vi "Example.vi"() -> ()   [LabVIEW 2018]
uses:
  Data Def/IT8800-Setting.ctl
panel:
  in  "Range Type":u16(ring) items=["Current", "Voltage", "Power", "Conductance"]
  out "Range":u16(ring)=2 items=["Low", "Medium", "High"]
  in  "Tracer":bool
  in  "Apply":bool
  in  "Value":dbl=5.0
  in  "Operation Mode":enum16{"CC", "CV", "CP"}(ring)
  out "Input?":bool
  in  "Stop Load":bool
  in  "Apply Load":bool
  out "Chart":T1(graph)={"Voltage (Volts)"=-1.0, "Power (Watts)"=-1.0, "Current (Amps)"=-1.0}
  out "Stop?":bool
  in  "IT8800 Setting In In":T2={"VISA Resource Name"="COM4", "Baud Rate"=9600, "Stop Bits"=10, "Wait For Read(ms)"=10} {"Stop Bits" items=["1.0"=10, "2.0"=20]; "Baud Rate" items=["2400"=2400, "4800"=4800, "9600"=9600, "19200"=19200]}
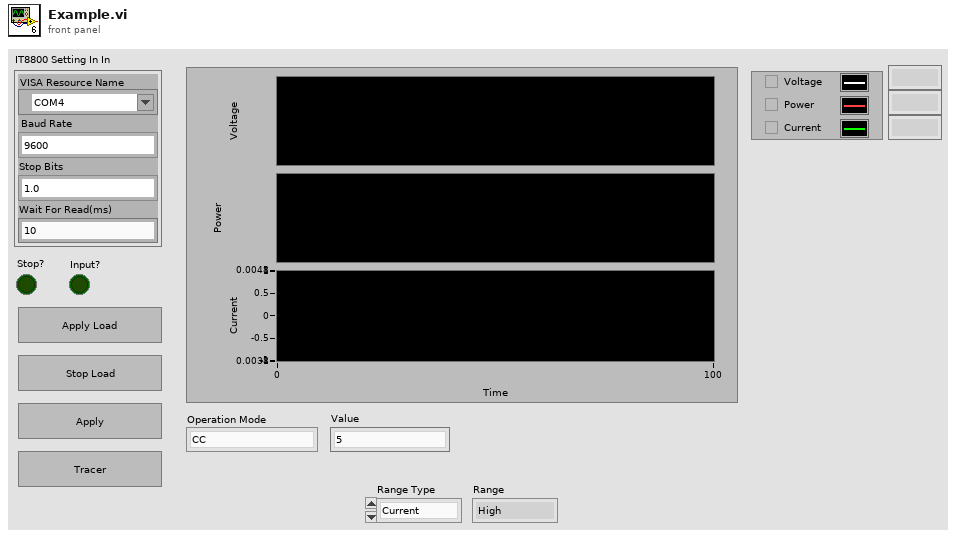
[diagram p1: front panel]
types:
  T1 = cluster{"Voltage (Volts)":dbl, "Power (Watts)":dbl, "Current (Amps)":dbl}
  T2 = typedef "IT8800-Setting.ctl" = cluster{"VISA Resource Name":refnum<visa-resource-name>, "Baud Rate":u32, "Stop Bits":u16, "Wait For Read(ms)":u32}
  T3 = typedef "IT8800-Measurement Data.ctl" = cluster{"Current (Amps)":dbl, "Power (Watts)":dbl, "Voltage (Volts)":dbl, "Elapsed Time (Sec) ":dbl}
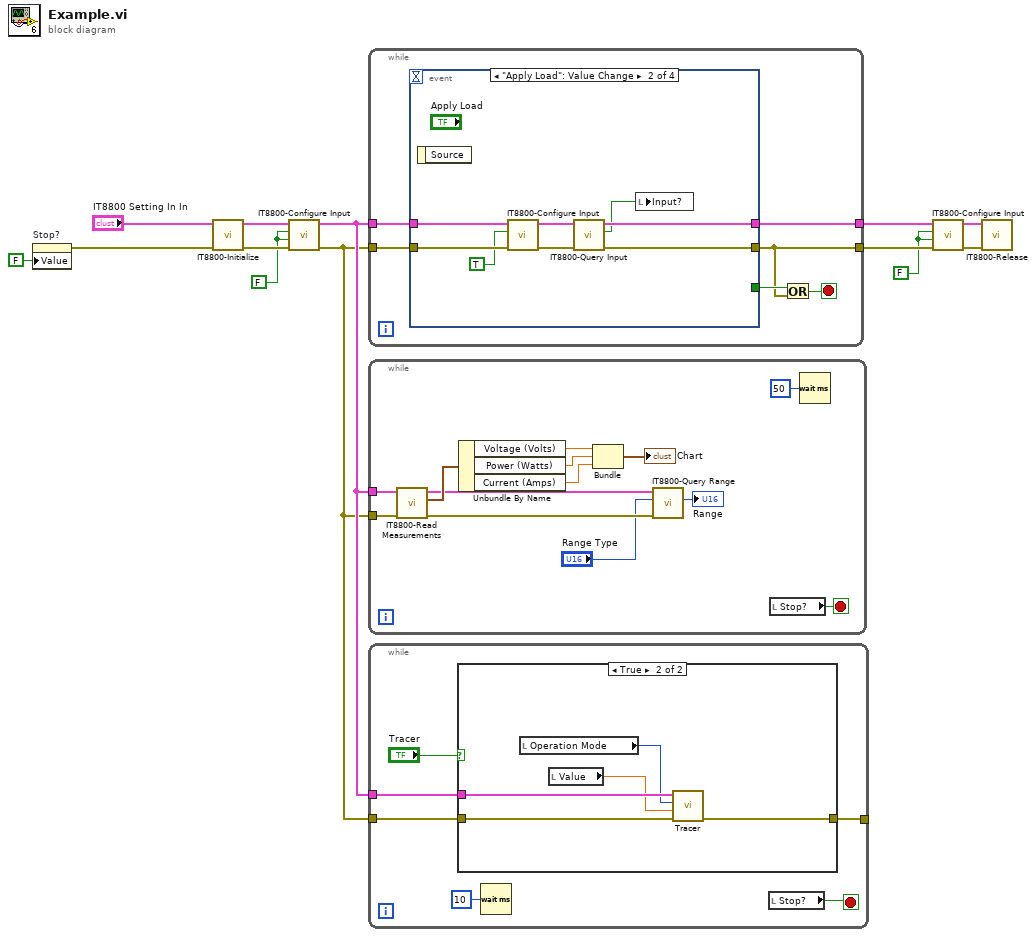
[diagram p0: block diagram]
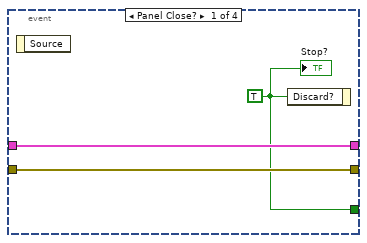
[diagram p3: hidden frame]
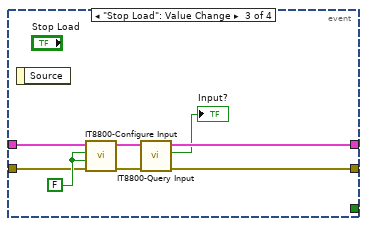
[diagram p4: hidden frame]
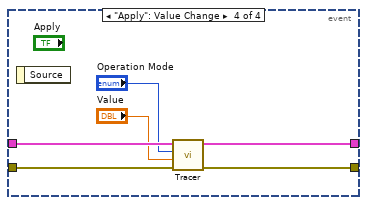
[diagram p5: hidden frame]
diagram:
  w5 = FALSE ("Enable Input")
  w10 = FALSE ("Enable Input")
  n1 = property on="Stop?" class="Bool (strict)"("Value"=FALSE ("Stop?")) -> (error out=w4:errorcluster)  [unwired: 2 in, 1 out]
  n2 = call "IT8800-Initialize.vi"("error in (no error)"=w4, "ITech Setting In"="IT8800 Setting In In") -> ("error out"=w11:errorcluster, "IT8800 Setting In Out"=w12:T2)  [unwired: 8 in]
  n3 = call "IT8800-Configure Input.vi"("error in"=w11, "Enable Input Short"=w10, "Enable Input"=w10, "IT8800 Setting In In"=w12) -> ("error out"=w1:errorcluster, "IT8800 Setting In Out"=w2:T2)  [unwired: 6 in]
  n4 = while {
    tunnel: w2 -> [w18]
    tunnel: w1 -> [w19]
    tunnel: [w16] -> w8
    tunnel: [w14] -> w9
    stop <- w15 stop-if-true
    n5 = event shown="[1] \"Apply Load\": Value Change" {
      selector: _ -> [_ _ _ _]
      dyn-events: _ -> [_ _ _ _]
      timeout: _ -> [_ _ _ _]
      tunnel: w19 -> [w22 w29 w36 w43]
      tunnel: w18 -> [w21 w30 w37 w44]
      tunnel: [w22 w25 w33 w42] -> w16
      tunnel: [w20 _ _ _] -> w17
      tunnel: [w21 w24 w32 w41] -> w14
      event Panel Close? {
        w20 = TRUE ("Discard?")
        n6 = event-data() -> ()  [unwired: 1 in, 1 out]
        n7 = event-data("Discard?"=w20) -> ()  [unwired: 1 in, 1 out]
        "Stop?" <- w20
      }
      event "Apply Load": Value Change {
        n8 = event-data() -> ()  [unwired: 1 in, 1 out]
        n9 = call "IT8800-Configure Input.vi"("error in"=w29, "Enable Input"=TRUE, "IT8800 Setting In In"=w30) -> ("error out"=w26:errorcluster, "IT8800 Setting In Out"=w27:T2)  [unwired: 7 in]
        n10 = call "IT8800-Query Input.vi"("error in"=w26, "IT8800 Setting In In"=w27) -> ("error out"=w25:errorcluster, "Input?"=w23:bool, "IT8800 Setting In Out"=w24:T2)  [unwired: 7 in]
        n11 = local write "Input?"(w23) -> ()
      }
      event "Stop Load": Value Change {
        w38 = FALSE ("Enable Input")
        n12 = event-data() -> ()  [unwired: 1 in, 1 out]
        n13 = call "IT8800-Configure Input.vi"("error in"=w36, "Enable Input Short"=w38, "Enable Input"=w38, "IT8800 Setting In In"=w37) -> ("error out"=w34:errorcluster, "IT8800 Setting In Out"=w35:T2)  [unwired: 6 in]
        n14 = call "IT8800-Query Input.vi"("error in"=w34, "IT8800 Setting In In"=w35) -> ("error out"=w33:errorcluster, "Input?"=→"Input?":bool, "IT8800 Setting In Out"=w32:T2)  [unwired: 7 in]
      }
      event "Apply": Value Change {
        n15 = event-data() -> ()  [unwired: 1 in, 1 out]
        n16 = call "Tracer.vi"("error in"=w43, "Value"="Value", "Operation Mode"="Operation Mode", "IT8800 Setting In In"=w44) -> ("error out"=w42:errorcluster, "IT8800 Setting In Out"=w41:T2)  [unwired: 6 in]
      }
    }
    n17 = Or(x=w17, y=w16) -> (x .or. y?=w15:bool)
  }
  n18 = while {
    tunnel: w2 -> [w55]
    tunnel: w1 -> [w56]
    stop <- w57 stop-if-true
    n19 = call "IT8800-Read Measurements.vi"("error in"=w56, "IT8800 Setting In In"=w55) -> ("error out"=w48:errorcluster, "Measurement Data"=w54:T3, "IT8800 Setting In Out"=w47:T2)  [unwired: 7 in]
    n20 = Unbundle By Name(w54) -> ("Voltage (Volts)"=w53:dbl, "Power (Watts)"=w52:dbl, "Current (Amps)"=w51:dbl)
    n21 = Bundle("Voltage (Volts)"=w53, "Power (Watts)"=w52, "Current (Amps)"=w51) -> (→"Chart":T1)  [unwired: 1 in]
    n22 = call "IT8800-Query Range.vi"("error in"=w48, "Range Type"="Range Type", "IT8800 Setting In In"=w47) -> ("Range"=→"Range":u16)  [unwired: 6 in, 2 out]
    n23 = local read "Stop?"() -> (w57:bool)
    n24 = Wait (ms)(milliseconds to wait=u32 50) -> ()  [unwired: 1 out]
  }
  n25 = while {
    tunnel: w2 -> [w60]
    tunnel: w1 -> [w59]
    tunnel: [w58] -> _
    stop <- w63 stop-if-true
    n26 = case shown="True" "Tracer" {
      tunnel: w60 -> [_ w69]
      tunnel: w59 -> [w64 w68]
      tunnel: [w64 w67] -> w58
      frame False {
      }
      frame True {
        n27 = local read "Operation Mode"() -> (w66:enum16{"CC", "CV", "CP"})
        n28 = local read "Value"() -> (w65:dbl)
        n29 = call "Tracer.vi"("error in"=w68, "Value"=w65, "Operation Mode"=w66, "IT8800 Setting In In"=w69) -> ("error out"=w67:errorcluster)  [unwired: 6 in, 1 out]
      }
    }
    n30 = Wait (ms)(milliseconds to wait=u32 10) -> ()  [unwired: 1 out]
    n31 = local read "Stop?"() -> (w63:bool)
  }
  n32 = call "IT8800-Configure Input.vi"("error in"=w8, "Enable Input Short"=w5, "Enable Input"=w5, "IT8800 Setting In In"=w9) -> ("error out"=w6:errorcluster, "IT8800 Setting In Out"=w7:T2)  [unwired: 6 in]
  n33 = call "IT8800-Release.vi"("error in"=w6, "IT8800 Setting In"=w7) -> ()  [unwired: 9 in, 1 out]
